vi "testBenchmarkSystemDefinitionPasses.vi"(8 "error in (no error)":errorcluster, 11 "TestCase in":refnum<class "VeriStandTestCaseSystemTests.lvclass">) -> (0 "error out":errorcluster, 3 "TestCase out":refnum<class "VeriStandTestCaseSystemTests.lvclass">)   [LabVIEW 2027, in "VeriStandTestCaseSystemTests.lvclass"]
uses:
  VeriStandTestCaseSystemTests.lvclass
  Source/VeriStandTestCase/VeriStandTestCase.lvclass
  C:/Program Files/National Instruments/LabVIEW 2027/vi.lib/addons/_JKI Toolkits/VI Tester/TestCase.llb/TestCase.lvclass
  <vilib>/addons/_JKI Toolkits/VI Tester/TestCase.llb/TestCase.lvclass
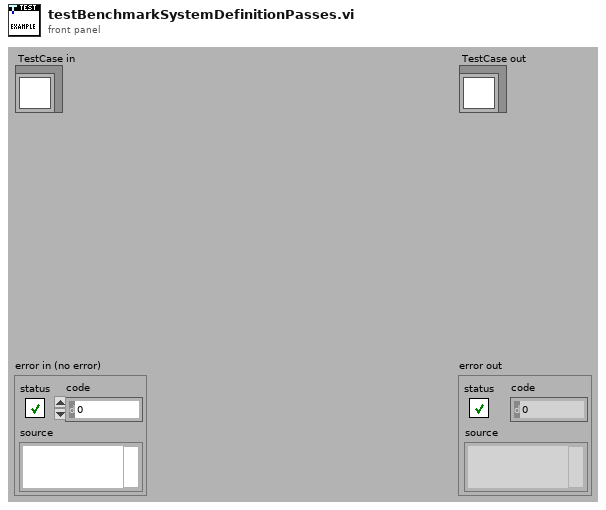
[diagram p1: front panel]
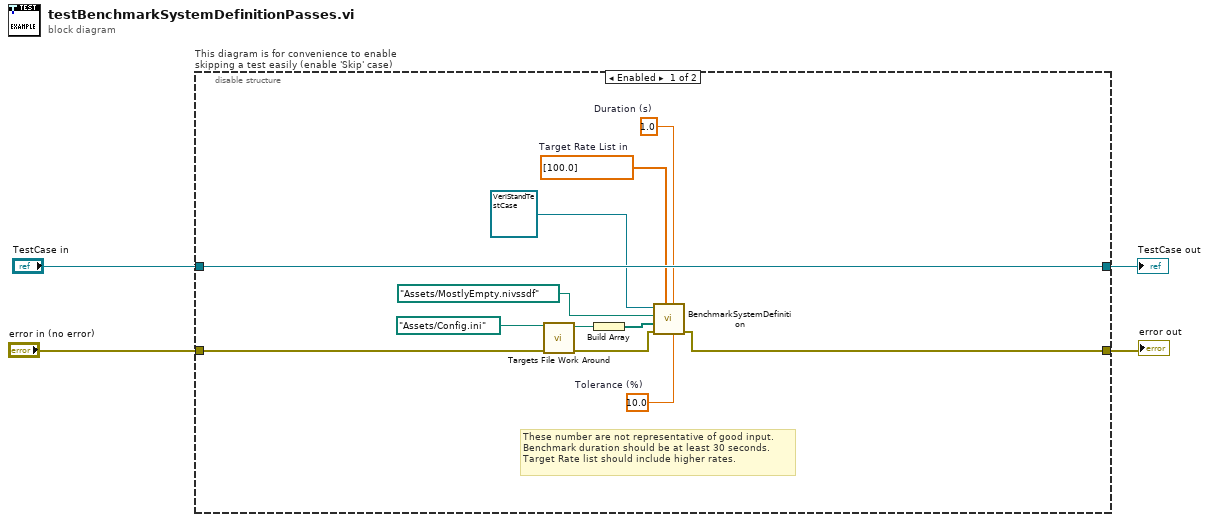
[diagram p0: block diagram]
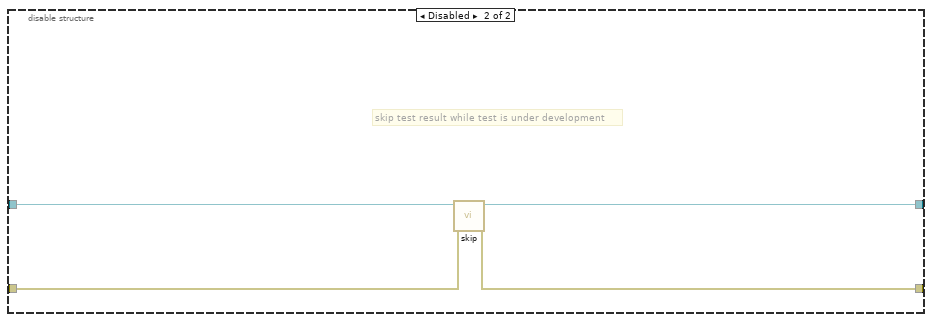
[diagram p2: hidden frame]
diagram:
  n1 = disable-structure "This diagram is for convenience to enable skipping a test easily (enable 'Skip' case)" shown="Enabled" {
    disable-tunnel: "TestCase in" -> [w16 w20]
    disable-tunnel: [w16 w18] -> w1
    disable-tunnel: [w14 w19] -> w3
    disable-tunnel: "error in (no error)" -> [w15 w17]
    frame Enabled {
      w9 = 10.0  # Tolerance (%)
      w10 = 1.0  # Duration (s)
      w11 = dbl[] [100.0]  # Target Rate List in
      # "These number are not representative of good input.\nBenchmark duration should be at least 30 seconds.\nTarget Rate list should include higher rates."
      n2 = call "Targets File Work Around.vi"("error in (no error)"=w15, "overrides file in"=path "Assets/Config.ini" ("overrides files")) -> ("error out"=w8:errorcluster, "overrides file out"=w6:path)  [unwired: 8 in]
      n3 = Build Array(w6) -> (w5:path[])
      n4 = call-dynamic "BenchmarkSystemDefinition.vi"("Tolerance (%)"=w9, "Duration (s)"=w10, "Target Rate List in"=w11, "error in (no error)"=w8, "overrides files"=w5, "System Definition File"=path "Assets/MostlyEmpty.nivssdf", "VeriStandTestCase in"=refnum<class "VeriStandTestCase.lvclass"> refnum ("VeriStand Test Case in")) -> ("error out"=w14:errorcluster)  [unwired: 3 in, 1 out]
    }
    frame Disabled {
      # "skip test result while test is under development"
      n5 = call <vilib>:"skip.vi"("error in (no error)"=w17, "TestCase in"=w20) -> ("error out"=w19:errorcluster, "TestCase out"=w18:refnum<class "VeriStandTestCaseSystemTests.lvclass">)  [unwired: 8 in]
    }
  }
  "error out" <- w3
  "TestCase out" <- w1
